vi "SetDataFolder.vi"(0 "User Data Folder":path, 2 "JustKillAllSavedReferences(False)":bool, 5 "error in (no error)":errorcluster, 8 "Webview container":refnum<k24>) -> (14 "Environment":refnum<k24>, 15 "UserDataFolder":string="C:\\ProgramData\\LcWebVIEW", 16 "Error Message":string, 19 "error out":errorcluster)   [LabVIEW 2018, in "LcWebView.lvclass"]
uses:
  LcWebView.lvclass
  C:/Projects/LcWebView2/LcWebView/LcWebView_class/data/Microsoft.Web.WebView2.Core.dll
  data/Microsoft.Web.WebView2.Core.dll
  C:/Projects/LcWebView2/LcWebView/LcWebView_class/data/Microsoft.Web.WebView2.WinForms.dll
  data/Microsoft.Web.WebView2.WinForms.dll
  <vilib>/Utility/sysdir.llb/System Directory Type.ctl
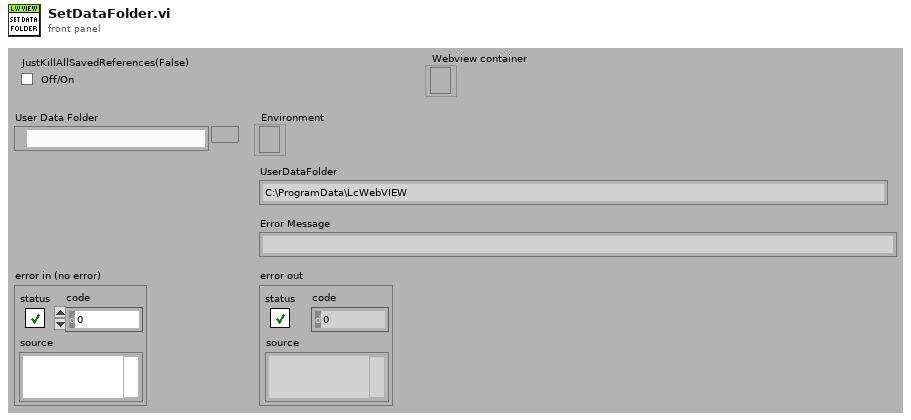
[diagram p1: front panel]
types:
  T1 = typedef "System Directory Type.ctl" = i32
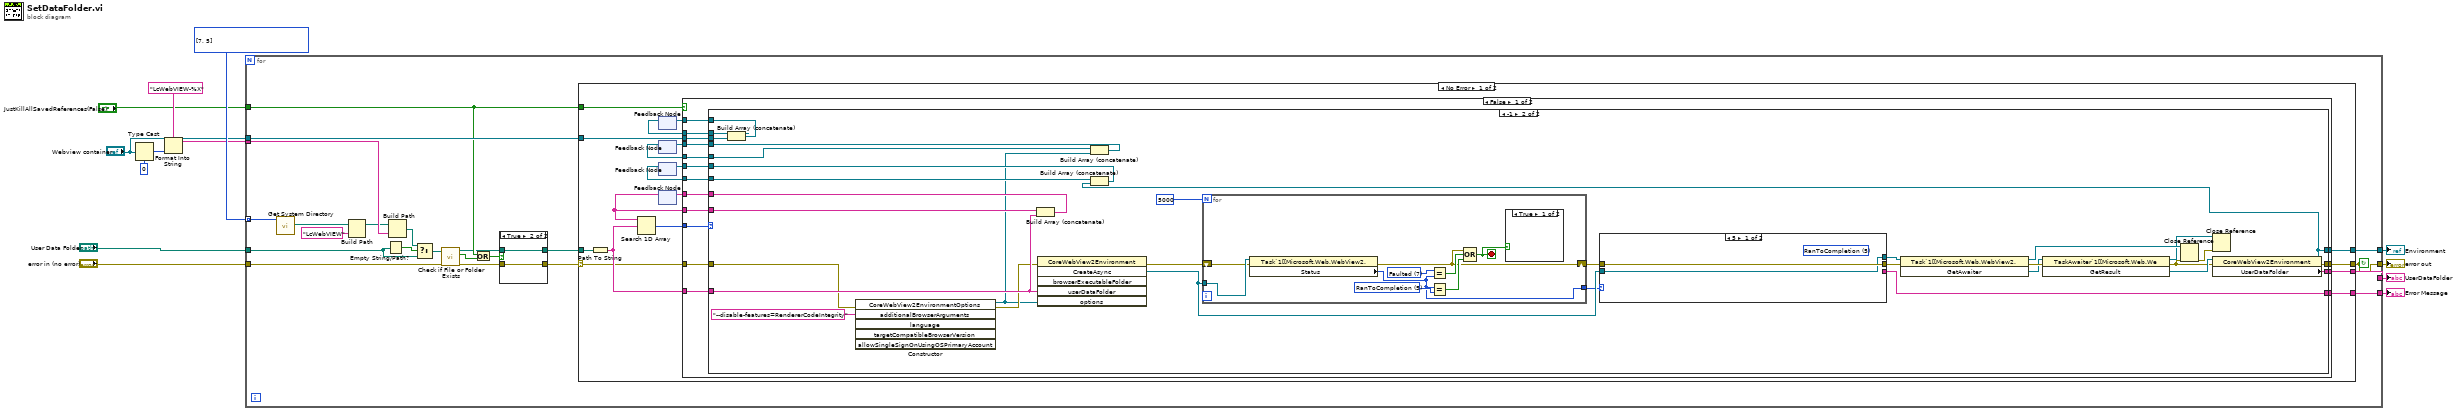
[diagram p0: block diagram]
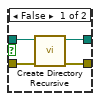
[diagram p2: hidden frame]
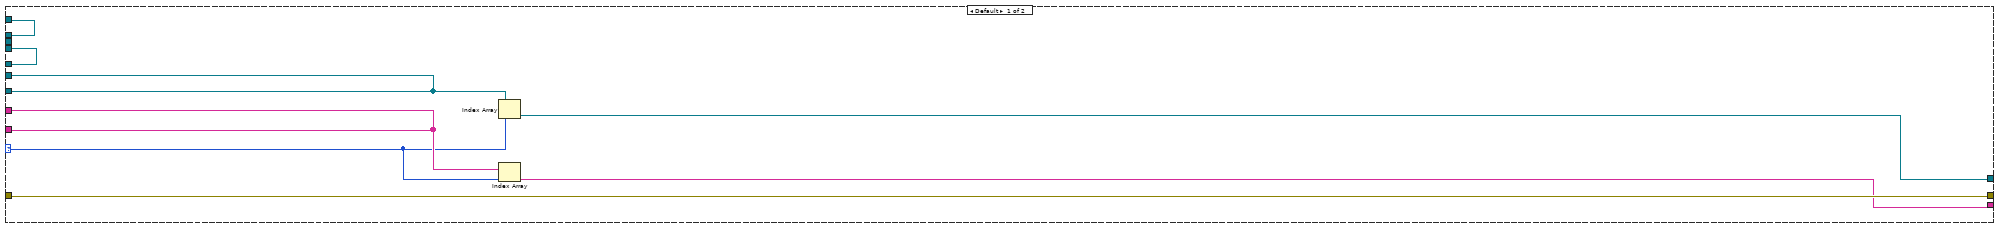
[diagram p3: hidden frame]
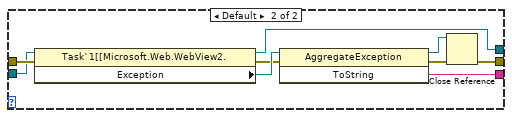
[diagram p4: hidden frame]
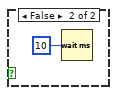
[diagram p5: hidden frame]
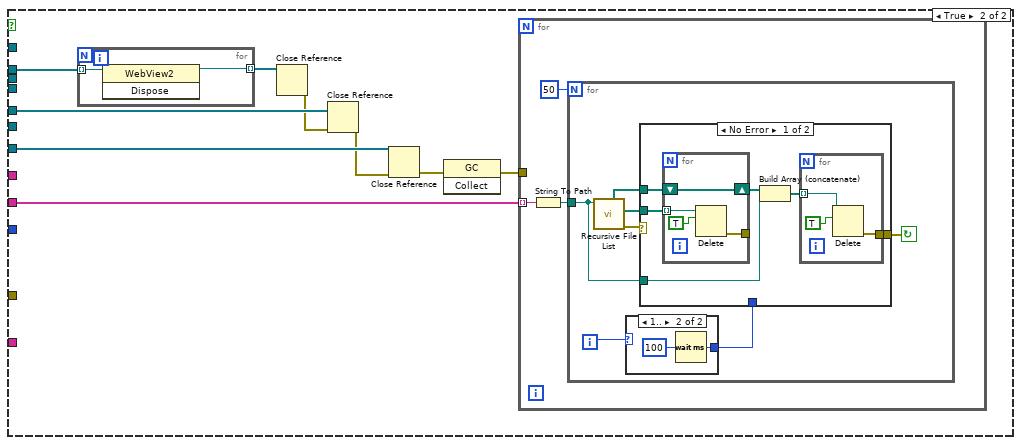
[diagram p6: hidden frame]
diagram:
  w13 = T1[] [7, 5] items=["User Home"=0, "User Desktop"=1, "User Documents"=2, "User Application Data"=3, "User Preferences"=4, "User Temporary"=5, "Public Documents"=6, "Public Application Data"=7, "Public Preferences"=8, "Public Cache"=13, "System Core Libraries"=9, "System Installed Libraries"=10, "Application Files"=11, "Boot Volume Root"=12] ("Array")
  n1 = Type Cast(type=u32 0 ("WebView2Control ID"), x="Webview container") -> (*(type *) &x=w3:u32)
  n2 = Format Into String(format string="LcWebVIEW-%X", w3) -> (resulting string=w5:string)  [unwired: 2 in, 1 out]
  n3 = for {
    tunnel: w13 -> [w35] mode=indexing
    tunnel: [w32] -> w10
    tunnel: [w31] -> w9
    tunnel: [w30] -> w8
    tunnel: "User Data Folder" -> [w29]
    tunnel: w5 -> [w28]
    tunnel: "Webview container" -> [w27]
    tunnel: "JustKillAllSavedReferences(False)" -> [w26]
    tunnel: "error in (no error)" -> [w34]
    tunnel: [w24] -> w11
    stop <- w24 continue-if-true
    n4 = call <vilib>:"Get System Directory.vi"("system directory type"=w35) -> ("system directory"=w17:path)  [unwired: 10 in]
    n5 = Build Path(base path=w17, name or relative path="LcWebVIEW") -> (appended path=w16:path)
    n6 = Empty String/Path?(string/path=w29) -> (empty?=w20:bool)
    n7 = Build Path(base path=w16, name or relative path=w28) -> (appended path=w19:path)
    n8 = Select(t=w19, s=w20, f=w29) -> (s? t:f=w18:path)
    n9 = call <vilib>:"Check if File or Folder Exists.vi"("error in (no error)"=w34, "path"=w18) -> ("error out"=w23:errorcluster, "file or folder exists?"=w21:bool, "dup path"=w22:path)  [unwired: 7 in]
    n10 = Or(x=w26, y=w21) -> (x .or. y?=w14:bool)
    n11 = case shown="True" w14 {
      tunnel: w22 -> [w39 w40]
      tunnel: w23 -> [w38 w41]
      tunnel: [w37 w41] -> w25
      tunnel: [w36 w40] -> w33
      frame False {
        n12 = call <vilib>:"Create Directory Recursive.vi"("error in (no error)"=w38, "directory"=w39) -> ("error out"=w37:errorcluster, "directory copy"=w36:path)  [unwired: 3 in, 1 out]
      }
      frame True {
      }
    }
    n13 = case shown="No Error" w25 {
      selector: w25 -> [w42 w173]
      tunnel: w33 -> [w59 _]
      tunnel: [w57 w173] -> w24
      tunnel: [w58 _] -> w32
      tunnel: [w55 _] -> w31
      tunnel: [w56 _] -> w30
      tunnel: w26 -> [w46 _]
      tunnel: w27 -> [w43 _]
      frame No Error {
        n14 = Path To String(path=w59) -> (string=w54:string)
        n15 = feedback #1() -> (w44:refnum<k24>[])  [unwired: 1 in]
        n16 = feedback #2() -> (w47:refnum<k24>[])  [unwired: 1 in]
        n17 = feedback #3() -> (w50:refnum<k24>[])  [unwired: 1 in]
        n18 = feedback #4() -> (w52:string[])  [unwired: 1 in]
        n19 = Search 1D Array(1D array=w52, element=w54) -> (index of element=w53:i32)  [unwired: 1 in]
        n20 = case shown="False" w46 {
          tunnel: w42 -> [w75 _]
          tunnel: [w74 _] -> w58
          tunnel: [w73 _] -> w57
          tunnel: [w72 _] -> w56
          tunnel: [w71 _] -> w55
          tunnel: w54 -> [w70 _]
          tunnel: w53 -> [w69 _]
          tunnel: w52 -> [w68 w140]
          tunnel: [w67 _] -> w51
          tunnel: w50 -> [w66 w145]
          tunnel: [w65 _] -> w49
          tunnel: [w64 _] -> w48
          tunnel: w47 -> [w63 w144]
          tunnel: [w61 _] -> w45
          tunnel: w44 -> [w62 w143]
          tunnel: w43 -> [w60 _]
          frame False {
            n21 = case shown="-1" w69 {
              selector: w69 -> [w79 _]
              tunnel: w75 -> [w81 w92]
              tunnel: [w78 w115] -> w74
              tunnel: [w81 w108] -> w73
              tunnel: [w82 w91] -> w72
              tunnel: [_ w106] -> w71
              tunnel: w70 -> [_ w98]
              tunnel: w68 -> [w80 w99]
              tunnel: [w80 w97] -> w67
              tunnel: w66 -> [w83 w96]
              tunnel: [w83 w95] -> w65
              tunnel: w63 -> [w77 w89]
              tunnel: [w77 w84] -> w64
              tunnel: w62 -> [w76 w87]
              tunnel: [w76 w85] -> w61
              tunnel: w60 -> [_ w86]
              frame Default {
                n22 = Index Array(array=w83, index=w79) -> (element=w82:refnum<k24>)
                n23 = Index Array(array=w80, index=w79) -> (element=w78:string)
              }
              frame -1 {
                n24 = Build Array (concatenate)(w87, w86) -> (w85:refnum<k24>[])
                n25 = constructor class="CoreWebView2EnvironmentOptions"(error in=w92, "additionalBrowserArguments"="--disable-features=RendererCodeIntegrity" ("AdditionalBrowserArguments")) -> (reference out=w90:refnum<k24>, error out=w93:errorcluster)  [unwired: 5 in, 5 out]
                n26 = Build Array (concatenate)(w99, w98) -> (w97:string[])
                n27 = invoke class="CoreWebView2Environment" method="CreateAsync"(error in=w93, "userDataFolder"=w98, "options"=w90) -> (error out=w88:errorcluster, "CreateAsync"=w104:refnum<k24>)  [unwired: 3 in, 4 out]
                n28 = Build Array (concatenate)(w89, w90) -> (w84:refnum<k24>[])
                n29 = for {
                  N: 5000 -> [_]
                  tunnel: w104 -> [w135]
                  shift-right: [w129] -> w107
                  shift-left: w88 -> [w134]
                  tunnel: [w128] -> w102
                  stop <- w127 stop-if-true
                  w132 = 5 items=["Created", "WaitingForActivation", "WaitingToRun", "Running", "WaitingForChildrenToComplete", "RanToCompletion", "Canceled", "Faulted"] ("Status")
                  w133 = 7 items=["Created", "WaitingForActivation", "WaitingToRun", "Running", "WaitingForChildrenToComplete", "RanToCompletion", "Canceled", "Faulted"] ("Status")
                  n30 = property class="Task`1[[Microsoft.Web.WebView2."(reference=w135, error in=w134) -> (error out=w129:errorcluster, "Status"=w128:i32)  [unwired: 1 out]
                  n31 = Equal?(x=w133, y=w128) -> (x = y?=w131:bool)
                  n32 = Equal?(x=w128, y=w132) -> (x = y?=w130:bool)
                  n33 = Compound Arithmetic op=OR(w129, w131, w130) -> (w127:bool)
                  n34 = case shown="True" w127 {
                    frame True {
                    }
                    frame False {
                      n35 = Wait (ms)(milliseconds to wait=u32 10) -> ()  [unwired: 1 out]
                    }
                  }
                }
                n36 = case shown="5" w102 {
                  tunnel: w107 -> [w117 w126]
                  tunnel: [_ w125] -> w106
                  tunnel: [w117 w118] -> w105
                  tunnel: w104 -> [w116 w123]
                  tunnel: [w116 w122] -> w103
                  frame 5 {
                    (unwired) 5 items=["Created", "WaitingForActivation", "WaitingToRun", "Running", "WaitingForChildrenToComplete", "RanToCompletion", "Canceled", "Faulted"] ("Status")
                  }
                  frame Default {
                    n37 = property class="Task`1[[Microsoft.Web.WebView2."(reference=w123, error in=w126) -> (reference out=w122:refnum<k24>, error out=w119:errorcluster, "Exception"=w124:refnum<k24>)
                    n38 = invoke class="AggregateException" method="ToString"(reference=w124, error in=w119) -> (reference out=w121:refnum<k24>, error out=w120:errorcluster, "ToString"=w125:string)  [unwired: 1 in]
                    n39 = Close Reference(reference=w121, error in (no error)=w120) -> (error out=w118:errorcluster)
                  }
                }
                n40 = invoke class="Task`1[[Microsoft.Web.WebView2." method="GetAwaiter"(reference=w103, error in=w105) -> (reference out=w110:refnum<k24>, error out=w113:errorcluster, "GetAwaiter"=w111:refnum<k24>)  [unwired: 1 in]
                n41 = invoke class="TaskAwaiter`1[[Microsoft.Web.We" method="GetResult"(reference=w111, error in=w113) -> (reference out=w100:refnum<k24>, error out=w109:errorcluster, "GetResult"=w112:refnum<k24>)  [unwired: 1 in]
                n42 = Close Reference(reference=w110, error in (no error)=w109) -> (error out=w101:errorcluster)
                n43 = Close Reference(reference=w100, error in (no error)=w101) -> ()  [unwired: 1 out]
                n44 = property class="CoreWebView2Environment"(reference=w112, error in=w109) -> (reference out=w91:refnum<k24>, error out=w108:errorcluster, "UserDataFolder"=w115:string)
                n45 = Build Array (concatenate)(w96, w91) -> (w95:refnum<k24>[])
              }
            }
          }
          frame True {
            n46 = for {
              tunnel: w143 -> [w172] mode=indexing
              tunnel: [w171] -> w142 mode=indexing
              n47 = invoke class="WebView2" method="Dispose"(reference=w172) -> (reference out=w171:refnum<k24>)  [unwired: 2 in, 2 out]
            }
            n48 = Close Reference(reference=w142) -> (error out=w139:errorcluster)  [unwired: 1 in]
            n49 = Close Reference(reference=w144, error in (no error)=w139) -> (error out=w138:errorcluster)
            n50 = Close Reference(reference=w145, error in (no error)=w138) -> (error out=w137:errorcluster)
            n51 = invoke class="GC" method="Collect"(error in=w137) -> (error out=w141:errorcluster)  [unwired: 2 in, 2 out]
            n52 = for {
              tunnel: w141 -> [_]
              tunnel: w140 -> [w148] mode=indexing
              n53 = String To Path(string=w148) -> (path=w147:path)
              n54 = for {
                N: 50 -> [_]
                tunnel: w147 -> [w153]
                i -> [w150]
                stop <- w152 continue-if-true
                n55 = call <vilib>:"Recursive File List.vi"("Folder Path"=w153) -> ("error out"=w151:errorcluster, "All Files in Dir"=w155:path[], "All Folders"=w154:path[])  [unwired: 6 in, 2 out]
                n56 = case shown="1.." w150 {
                  tunnel: [_ w156] -> w149
                  frame 0, Default {
                  }
                  frame 1.. {
                    n57 = Wait (ms)(milliseconds to wait=u32 100) -> (millisecond timer value=w156:u32)
                  }
                }
                n58 = case shown="No Error" w151 {
                  tunnel: w155 -> [w163 _]
                  tunnel: w154 -> [w161 _]
                  tunnel: w153 -> [w159 _]
                  tunnel: [w158 _] -> w152
                  tunnel: w149 -> [_ _]
                  frame No Error {
                    n59 = for {
                      tunnel: w163 -> [w169] mode=indexing
                      tunnel: [w167] -> _
                      shift-right: [w168] -> w162
                      shift-left: w161 -> [w168]
                      n60 = Delete(path (use dialog)=w169, entire hierarchy (F)=TRUE) -> (error out=w167:errorcluster)  [unwired: 3 in, 2 out]
                    }
                    n61 = Build Array (concatenate)(w162, w159) -> (w160:path[])
                    n62 = for {
                      tunnel: w160 -> [w165] mode=indexing
                      tunnel: [w164] -> w158
                      n63 = Delete(path (use dialog)=w165, entire hierarchy (F)=TRUE) -> (error out=w164:errorcluster)  [unwired: 3 in, 2 out]
                    }
                  }
                  frame Error {
                    # "All files gone :-)"
                  }
                }
              }
            }
          }
        }
        n64 = feedback-in #1(w45) -> ()
        n65 = feedback-in #2(w48) -> ()
        n66 = feedback-in #3(w49) -> ()
        n67 = feedback-in #4(w51) -> ()
      }
      frame Error {
      }
    }
  }
  "error out" <- w11
  "UserDataFolder" <- w10
  "Error Message" <- w9
  "Environment" <- w8
